vi "Config File Path.vi"() -> (3 "appended path":path)   [LabVIEW 2015]
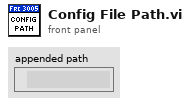
[diagram p1: front panel]
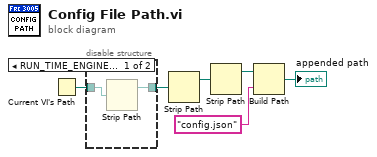
[diagram p0: block diagram]
diagram:
  n1 = Current VI's Path() -> (path=w6:path)
  n2 = disable-structure shown="RUN_TIME_ENGINE==True" {
    disable-tunnel: w6 -> [w8 w9]
    disable-tunnel: [w7 w9] -> w5
    frame condition #0 {
      n3 = Strip Path(path=w8) -> (stripped path=w7:path)  [unwired: 1 out]
    }
    frame condition #1 (active) {
    }
  }
  n4 = Strip Path(path=w5) -> (stripped path=w4:path)  [unwired: 1 out]
  n5 = Strip Path(path=w4) -> (stripped path=w1:path)  [unwired: 1 out]
  n6 = Build Path(base path=w1, name or relative path="config.json") -> (appended path=→"appended path":path)
